vi "数据表比对1表格对比.vi"(8 "error in (no error)":errorcluster, 9 "table输入 2":string(combo), 11 "table输入":string(combo)) -> (0 "error out":errorcluster, 2 "待发送第一条数据":string[](array[string]), 3 "待发送数据":string[][](table), 4 "获取有效数据":string[][](array[string]))   [LabVIEW 2016]
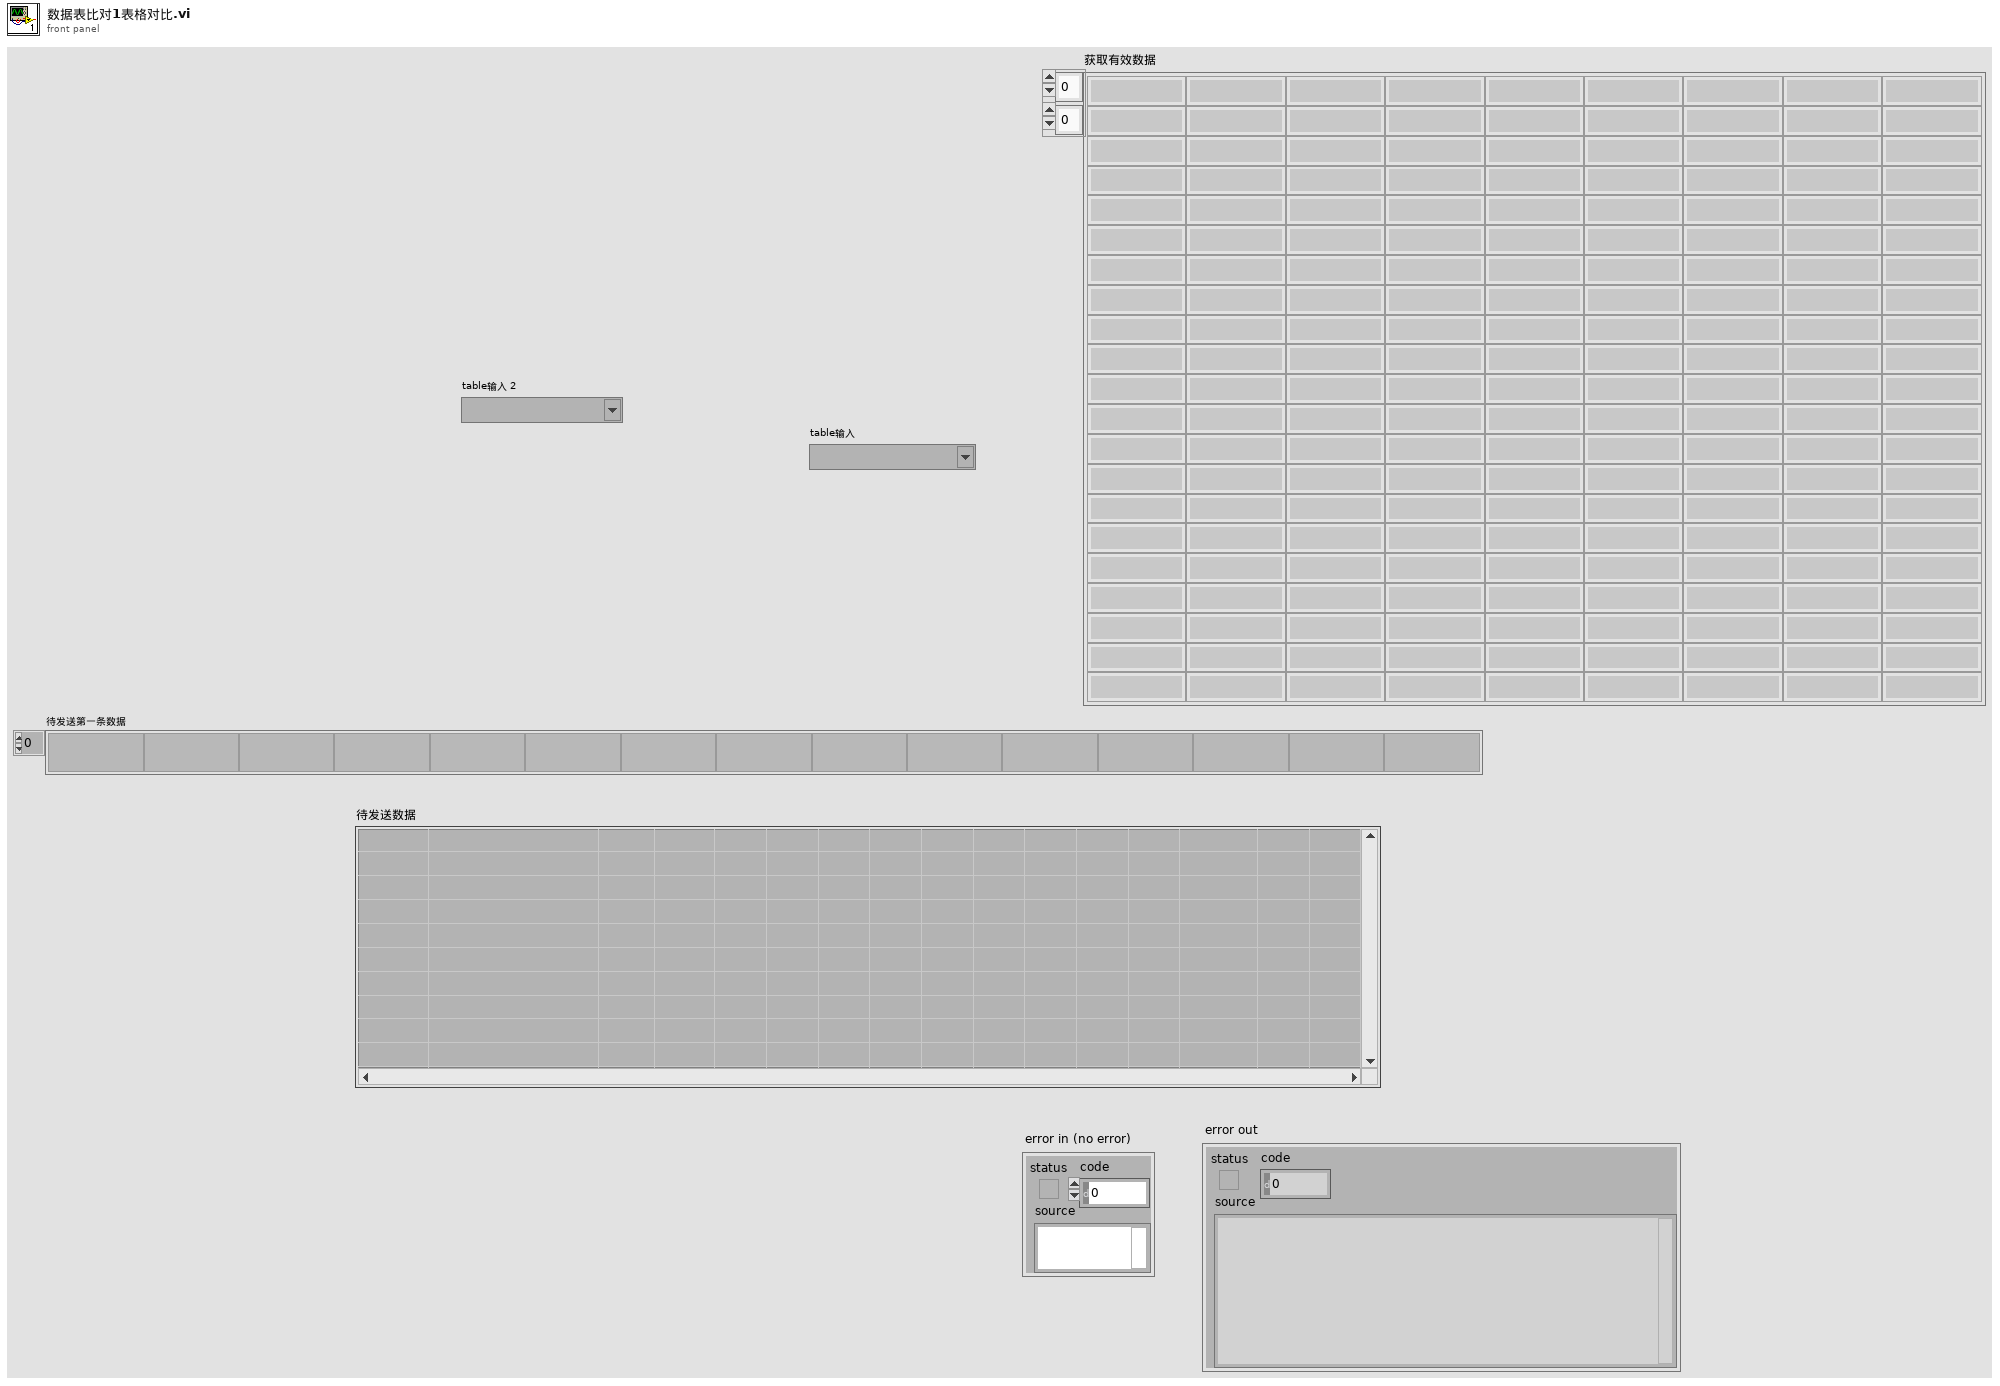
[diagram p1: front panel]
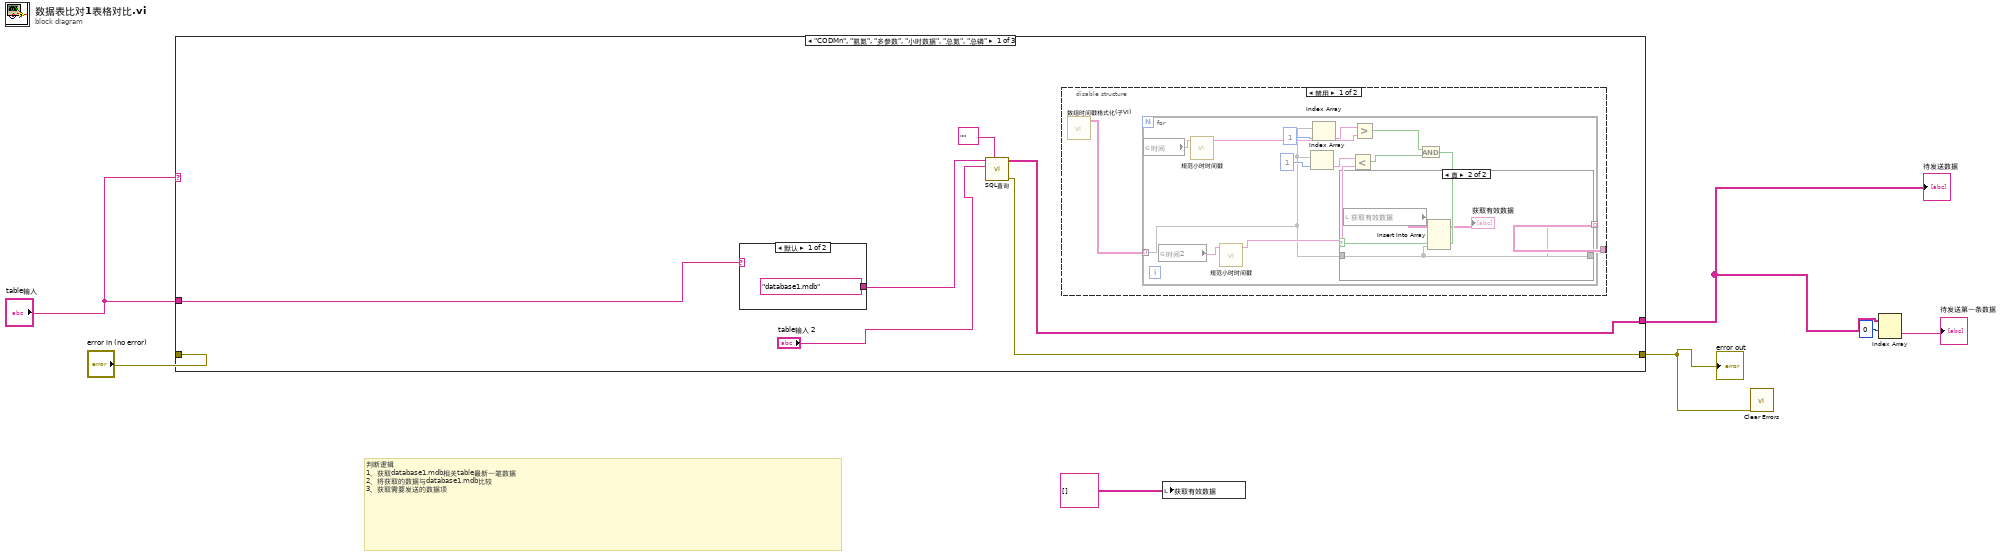
[diagram p0: block diagram]
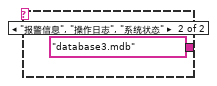
[diagram p4: hidden frame]
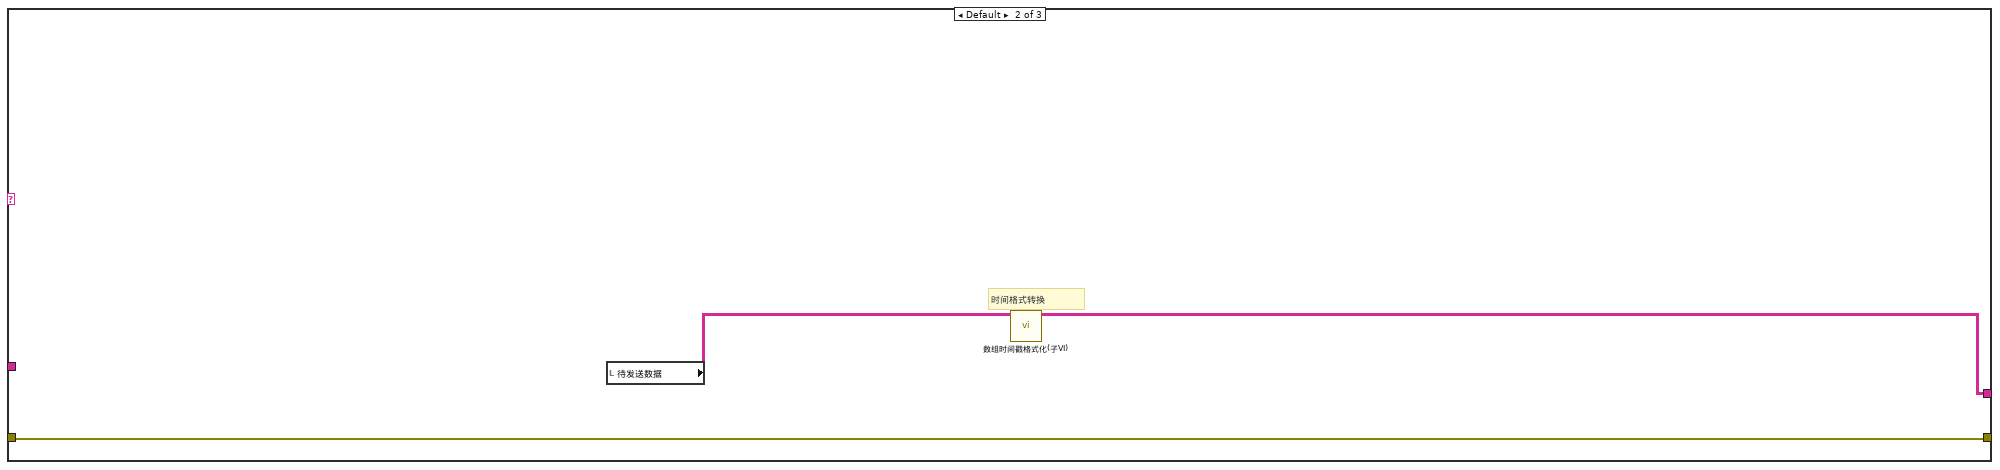
[diagram p5: hidden frame]
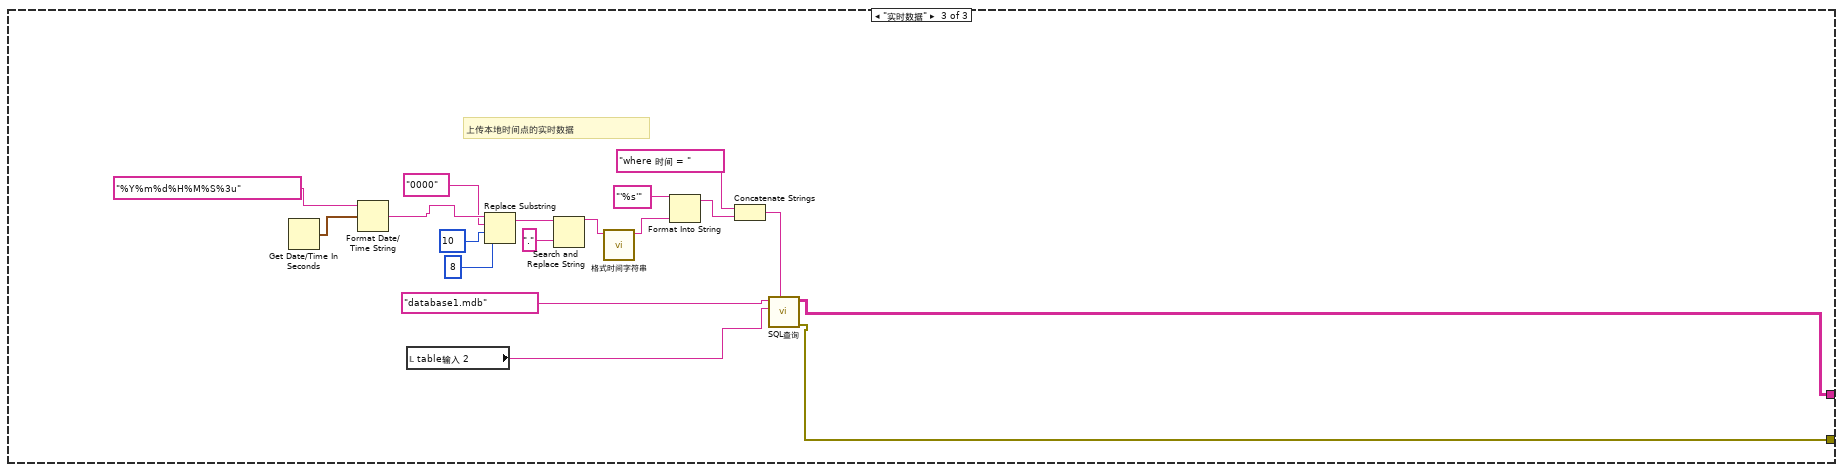
[diagram p6: hidden frame]
diagram:
  # "判断逻辑\n1、获取database1.mdb相关table最新一笔数据\n2、将获取的数据与database1.mdb比较\n3、获取需要发送的数据项"
  n1 = case shown="\"CODMn\", \"氨氮\", \"多参数\", \"小时数据\", \"总氮\", \"总磷\"" "table输入" {
    tunnel: "error in (no error)" -> [_ w36 _]
    tunnel: [w10 w36 w44] -> w5
    tunnel: [w9 w34 w45] -> w1
    tunnel: "table输入" -> [w13 _ _]
    frame "CODMn", "氨氮", "多参数", "小时数据", "总氮", "总磷" {
      n2 = case shown="默认" w13 {
        tunnel: ["database1.mdb" ("database") "database3.mdb" ("database")] -> w12
        frame Default {
        }
        frame "报警信息", "操作日志", "系统状态" {
        }
      }
      n3 = call "SQL查询.vi"("condition"="", "table输入"="table输入 2", "database"=w12) -> ("error out"=w10:errorcluster, "data"=w9:string[][])  [unwired: 7 in]
      n4 = disable-structure shown="禁用" {
        disable-tunnel: [w14 _] -> _
        frame Disabled {
          n5 = call "数组时间戳格式化(子VI).vi"() -> ("待发送数据输出"=w15:string[][])  [unwired: 11 in]
          n6 = for {
            tunnel: w15 -> [w16] mode=indexing
            tunnel: [w18] -> w14 mode=indexing
            n7 = global read "全局 时间.vi" "时间"() -> (w22:string)
            n8 = global read "全局 时间2.vi" "时间2"() -> (w20:string)
            n9 = call "规范小时时间戳.vi"("字符串"=w22) -> ("result string"=w21:string)  [unwired: 10 in]
            n10 = call "规范小时时间戳.vi"("字符串"=w20) -> ("result string"=w19:string)  [unwired: 10 in]
            n11 = Index Array(array=w16, index=1 ("索引")) -> (element=w25:string)
            n12 = Index Array(array=w16, index=1 ("索引")) -> (element=w27:string)
            n13 = Less?(x=w25, y=w19) -> (x < y?=w24:bool)
            n14 = Greater?(x=w27, y=w21) -> (0:w23:bool)
            n15 = And(x=w23, y=w24) -> (x .and. y?=w17:bool)
            n16 = case shown="真" w17 {
              tunnel: w16 -> [_ w31]
              tunnel: [_ w31] -> w18
              frame False {
              }
              frame True {
                n17 = local read "获取有效数据"() -> (w30:string[][])
                n18 = Insert Into Array(array=w30, new element=w31) -> (→"获取有效数据":string[][])  [unwired: 2 in]
              }
            }
          }
        }
        frame Enabled {
        }
      }
    }
    frame Default {
      # "时间格式转换"
      n19 = local read "待发送数据"() -> (w35:string[][])
      n20 = call "数组时间戳格式化(子VI).vi"("待发送数据输入"=w35) -> ("待发送数据输出"=w34:string[][])  [unwired: 10 in]
    }
    frame "实时数据" {
      # "上传本地时间点的实时数据"
      n21 = Get Date/Time In Seconds() -> (seconds since 1Jan1904=w50:timestamp)
      n22 = Format Date/Time String(time format string (%c)="%Y%m%d%H%M%S%3u" ("时间格式字符串(%c)"), seconds (now)=w50) -> (date/time string=w43:string)  [unwired: 1 in]
      n23 = local read "table输入 2"() -> (w46:string)
      n24 = Replace Substring(2:8 ("长度（子字符串长度）"), 3:10 ("偏移量(0)"), 4:"0000" ("子字符串(\"\")"), 5:w43) -> (1:w42:string)  [unwired: 1 out]
      n25 = Search and Replace String(input string=w42, search string="." ("搜索字符串")) -> (result string=w38:string)  [unwired: 6 in, 3 out]
      n26 = call "格式时间字符串.vi"("字符串"=w38) -> ("连接的字符串"=w37:string)  [unwired: 10 in]
      n27 = Format Into String(format string="'%s'" ("初始字符串"), w37) -> (resulting string=w53:string)  [unwired: 2 in, 1 out]
      n28 = Concatenate Strings("where 时间 = " ("condition"), w53) -> (w48:string)
      n29 = call "SQL查询.vi"("condition"=w48, "table输入"=w46, "database"="database1.mdb") -> ("error out"=w44:errorcluster, "data"=w45:string[][])  [unwired: 7 in]
    }
  }
  "待发送数据" <- w1
  "error out" <- w5
  n30 = local write "获取有效数据"(string[][] []) -> ()
  n31 = call <vilib>:"Clear Errors.vi"("error in (no error)"=w5) -> ()  [unwired: 5 in, 2 out]
  n32 = Index Array(array=w1, index (row)=0 ("索引 (行)")) -> (element=→"待发送第一条数据":string[])  [unwired: 1 in]
